vi "from string.vi"(8 "error in":errorcluster, 9 "data":string, 10 "version":string, 11 "user tag bus module configuration In":refnum<class "user tag bus module configuration.lvclass">) -> (0 "error out":errorcluster, 3 "user tag bus module configuration Out":refnum<class "user tag bus module configuration.lvclass">)   [LabVIEW 2013, in "user tag bus module configuration.lvclass"]
doc: "Provides an interface for loading a module configuration from a file or other serialized data source. It is recommended that all children of this class store data in two sets--data required for its own initialization, and any data required for parent initialization--and that each implementation uses the <b>Call Parent Method</b> primitive to de-serialize parent information. As a result, it is expected that every module configuration class calls <b>component configuration.lvclass:From String.vi</b>."
uses:
  user tag bus module configuration.lvclass
  state module configuration.ctl
  <vilib>/NI/Tag Bus Module Framework/channel/TBM channel.lvclass
  <vilib>/NI/Tag Bus Module Framework/module configuration/TBM module configuration.lvclass
  user tag bus module configuration.lvclass/user tag bus module configuration.ctl
  <vilib>/NI/Configuration Framework/serializable configuration/NISE_CEF_serializable configuration.lvclass
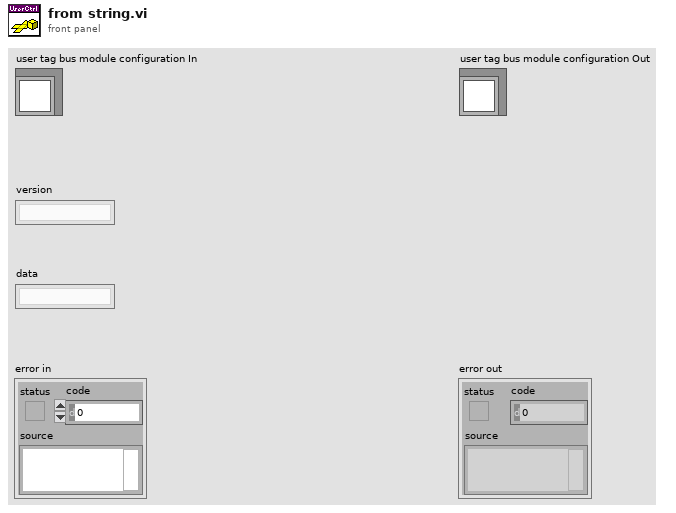
[diagram p1: front panel]
types:
  T1 = typedef "user tag bus module configuration.lvclass/state module configuration.ctl" = cluster{"fixed input":refnum<class "TBM channel.lvclass">, "fixed output":refnum<class "TBM channel.lvclass">, "initial state":u8}
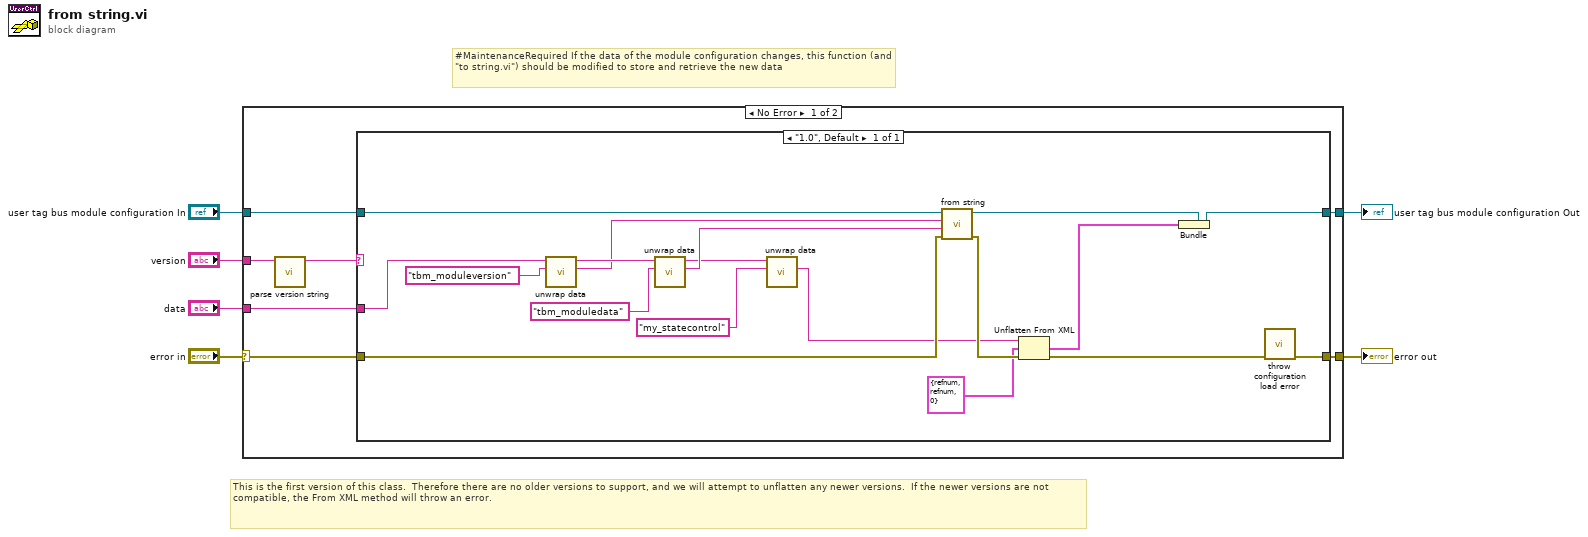
[diagram p0: block diagram]
diagram:
  # "#MaintenanceRequired If the data of the module configuration changes, this function (and \"to string.vi\") should be modified to store and retrieve the new data"
  # "This is the first version of this class.  Therefore there are no older versions to support, and we will attempt to unflatten any newer versions.  If the newer versions are not compatible, the From XML method will throw an error."
  n1 = case shown="No Error" "error in" {
    selector: "error in" -> [w7 w33]
    tunnel: "data" -> [w13 _]
    tunnel: "user tag bus module configuration In" -> [w12 w32]
    tunnel: [w11 w32] -> w5
    tunnel: [w10 w33] -> w4
    tunnel: "version" -> [w9 _]
    frame No Error {
      n2 = call <vilib>:"parse version string.vi"("full version"=w9) -> ("major.minor version"=w8:string)  [unwired: 7 in, 3 out]
      n3 = case shown="\"1.0\", Default" w8 {
        tunnel: w13 -> [w26]
        tunnel: w7 -> [w25]
        tunnel: w12 -> [w31]
        tunnel: [w20] -> w11
        tunnel: [w28] -> w10
        frame "1.0", Default {
          n4 = call <vilib>:"unwrap data.vi"("identifier"="tbm_moduleversion" ("additional identifier"), "data to unwrap"=w26) -> ("unwrapped data"=w21:string, "remaining string"=w27:string)  [unwired: 8 in]
          n5 = call <vilib>:"unwrap data.vi"("identifier"="tbm_moduledata" ("additional identifier"), "data to unwrap"=w27) -> ("unwrapped data"=w23:string, "remaining string"=w18:string)  [unwired: 8 in]
          n6 = call <vilib>:"unwrap data.vi"("identifier"="my_statecontrol" ("additional identifier"), "data to unwrap"=w18) -> ("unwrapped data"=w16:string)  [unwired: 8 in, 1 out]
          n7 = call-parent "from string.vi"("error in"=w25, "data"=w23, "version"=w21, "module configuration in"=w31) -> ("error out"=w29:errorcluster, "module configuration out"=w30:refnum<class "user tag bus module configuration.lvclass">)  [unwired: 6 in]
          n8 = Unflatten From XML(xml string=w16, type=T1 {"fixed input"=refnum, "fixed output"=refnum, "initial state"=0} ("state module configuration"), error in (no error)=w29) -> (value=w14:T1, error out=w19:errorcluster)
          n9 = Bundle(cluster=w30, w14) -> (w20:refnum<class "user tag bus module configuration.lvclass">)
          n10 = call <vilib>:"throw configuration load error.vi"("error in"=w19) -> ("error out"=w28:errorcluster)  [unwired: 10 in]
        }
      }
    }
    frame Error {
    }
  }
  "error out" <- w4
  "user tag bus module configuration Out" <- w5
